vi "Format Call Chain.vi"(5 "number of callers (-1: all)":i32=-1, 7 "delimiter (\" > \")":string=" > ", 9 "string length (-1: none)":i32=-1, 10 "remove namespaces? (T)":bool=TRUE, 11 "call chain":string[](array[string])) -> (3 "formatted call chain":string)   [LabVIEW 2018, in "GLog.lvlib" / "Format String.lvclass"]
uses:
  Format String.lvclass
  reuse_library/Utilities/Utilities.lvlib
panel:
  # "Connector Pane"
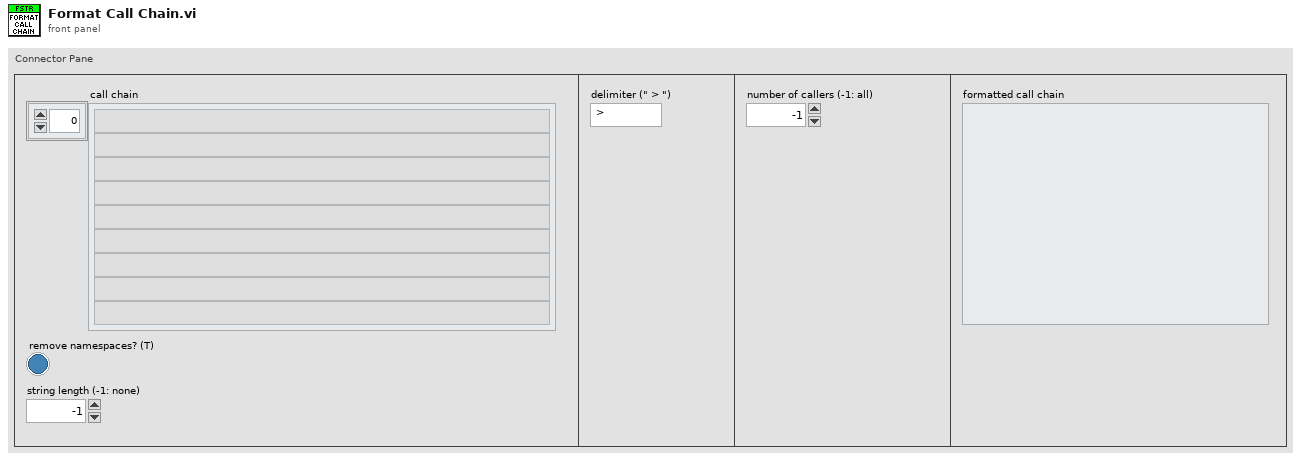
[diagram p1: front panel]
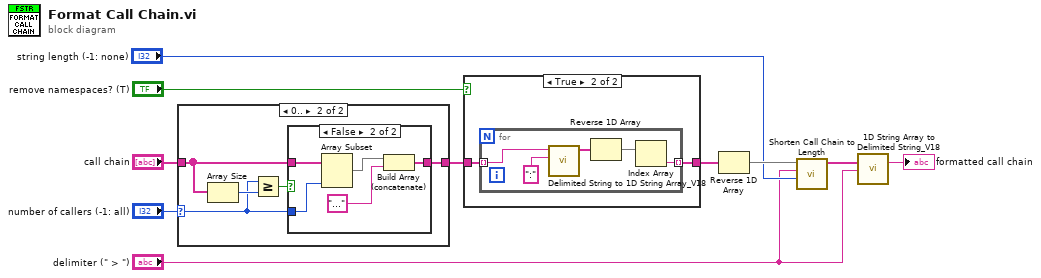
[diagram p0: block diagram]
diagram:
  n1 = case shown="0.." "number of callers (-1: all)" {
    selector: "number of callers (-1: all)" -> [_ w13]
    tunnel: "call chain" -> [w11 w15]
    tunnel: [w11 w16] -> w3
    frame ..-1 {
    }
    frame 0.. {
      n2 = Array Size(array=w15) -> (size(s)=w14:i32)
      n3 = Greater Or Equal?(x=w13, y=w14) -> (x >= y?=w12:bool)
      n4 = case shown="False" w12 {
        tunnel: [w17 w19] -> w16
        tunnel: w15 -> [w17 w21]
        tunnel: w13 -> [_ w20]
        frame True {
        }
        frame False {
          n5 = Array Subset(array=w21, length=w20) -> (w22:string[])  [unwired: 1 in]
          n6 = Build Array (concatenate)(w22, "…" ("String")) -> (w19:string[])
        }
      }
    }
  }
  n7 = case shown="True" "remove namespaces? (T)" {
    tunnel: w3 -> [w23 w25]
    tunnel: [w23 w24] -> w10
    frame False {
    }
    frame True {
      n8 = for {
        tunnel: w25 -> [w26] mode=indexing
        tunnel: [w27] -> w24 mode=indexing
        n9 = call "Delimited String to 1D String Array_V18.vi"("delimiter"=":", "delimited string"=w26) -> ("string array"=w29:string[])  [unwired: 9 in]
        n10 = Reverse 1D Array(array=w29) -> (reversed array=w28:string[])
        n11 = Index Array(array=w28) -> (element=w27:string)  [unwired: 1 in]
      }
    }
  }
  n12 = Reverse 1D Array(array=w10) -> (reversed array=w6:string[])
  n13 = call "Shorten Call Chain to Length.vi"("desired length"="string length (-1: none)", "delimiter"="delimiter (\" > \")", "call chain in"=w6) -> ("call chain out"=w7:string[])  [unwired: 8 in]
  n14 = call "1D String Array to Delimited String_V18.vi"("delimiter"="delimiter (\" > \")", "string array"=w7) -> ("delimited string"=→"formatted call chain":string)  [unwired: 9 in]
